vi "Arm Control.vi"(9 "Position":dbl, 10 "Arm Target":string) -> ()   [LabVIEW 2020]
uses:
  <vilib>/addons/control/pid/NI_PID_pid.lvlib
  <vilib>/addons/control/pid/pid.llb/PID (DBL).vi
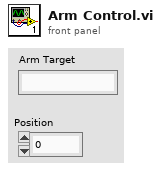
[diagram p1: front panel]
types:
  T1 = cluster{"proportional gain (Kc)":dbl, "integral time (Ti, min)":dbl, "derivative time (Td, min)":dbl}
  T2 = typedef "WPI_MotorControlDeviceRef.ctl" = cluster{"DeviceStatus":errorcluster, "Type":T3, "PWM":cluster{"PWM Channel":T4, "DeadBand":T5}, "CAN":cluster{"Device Number":u8, "SetOutput VI Ref":variant, "GetOutput VI Ref":variant, "Enable VI Ref":variant, "Disable VI Ref":variant, "Data":variant}, "Invert":bool, "DIO PWM":cluster{"PWM \"Enable\" Channel":T4, "DIOChannel":T6, "PWM Rate":dbl}}
  T3 = typedef "WPI_MotorControlType.ctl" = enum16{"PWM", "CAN", "DIO PWM"}
  T4 = typedef "FPGA_DIOPWMChannel.ctl" = enum8{"PWM 0", "PWM 1", "PWM 2", "PWM 3", "PWM 4", "PWM 5", "PWM 6", "PWM 7", "PWM 8", "PWM 9", "PWM MXP 0", "PWM MXP 1", "PWM MXP 2", "PWM MXP 3", "PWM MXP 4", "PWM MXP 5", "PWM MXP 6", "PWM MXP 7", "PWM MXP 8", "PWM MXP 9", "Invalid"}
  T5 = typedef "WPI_PWMDeadband.ctl" = cluster{"Name":string, "maxPositivePwm":i32, "minPositivePwm":i32, "centerPwm":i32, "maxNegativePwm":i32, "minNegativePwm":i32, "angularRange":u16}
  T6 = typedef "FPGA_DIOChannel.ctl" = enum8{"DIO 0", "DIO 1", "DIO 2", "DIO 3", "DIO 4", "DIO 5", "DIO 6", "DIO 7", "DIO 8", "DIO 9", "DIO MXP 0", "DIO MXP 1", "DIO MXP 2", "DIO MXP 3", "DIO MXP 4", "DIO MXP 5", "DIO MXP 6", "DIO MXP 7", "DIO MXP 8", "DIO MXP 9", "DIO MXP 10", "DIO MXP 11", "DIO MXP 12", "DIO MXP 13", "DIO MXP 14", "DIO MXP 15", "SPI Port CS1", "SPI Port CS2", "SPI Port CS3", "SPI Port MISO", "SPI Port MOSI", "Invalid"}
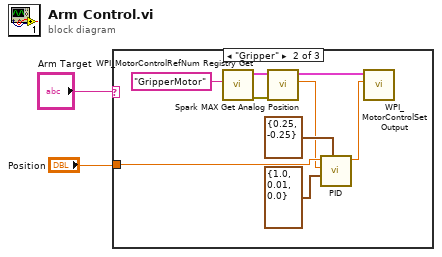
[diagram p0: block diagram]
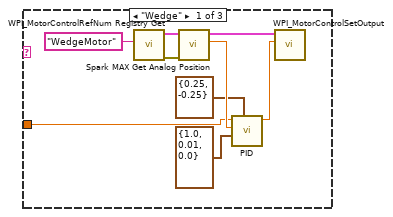
[diagram p2: hidden frame]
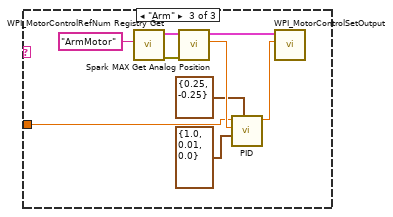
[diagram p3: hidden frame]
diagram:
  n1 = case shown="\"Gripper\"" "Arm Target" {
    tunnel: "Position" -> [w3 w20 w21]
    frame "Wedge" {
      n2 = call <vilib>:"WPI_MotorControlRefNum Registry Get.vi"("refnum name"="WedgeMotor") -> ("error out"=w8:errorcluster, "MotorControlDevRef"=w7:T2)  [unwired: 9 in]
      n3 = call <vilib>:"Spark MAX Get Analog Position.vi"("error in (no error)"=w8, "MotorControlDevRef in"=w7) -> ("Analog Position"=w9:dbl, "MotorControlDevRef out"=w10:T2)  [unwired: 6 in, 2 out]
      n4 = call-poly <vilib>:"PID.vi"("output range"=cluster{"output high":dbl, "output low":dbl} {"output high"=0.25, "output low"=-0.25}, "PID gains"=T1 {"proportional gain (Kc)"=1.0, "integral time (Ti, min)"=0.01, "derivative time (Td, min)"=0.0}, "process variable"=w9, "setpoint"=w3) -> ("output"=w11:dbl)  [unwired: 6 in, 1 out]
      n5 = call <vilib>:"WPI_MotorControlSetOutput.vi"("Output"=w11, "MotorControlDevRef"=w10) -> ()  [unwired: 7 in, 3 out]
    }
    frame "Gripper" {
      n6 = call <vilib>:"WPI_MotorControlRefNum Registry Get.vi"("refnum name"="GripperMotor") -> ("error out"=w15:errorcluster, "MotorControlDevRef"=w17:T2)  [unwired: 9 in]
      n7 = call <vilib>:"Spark MAX Get Analog Position.vi"("error in (no error)"=w15, "MotorControlDevRef in"=w17) -> ("Analog Position"=w14:dbl, "MotorControlDevRef out"=w13:T2)  [unwired: 6 in, 2 out]
      n8 = call-poly <vilib>:"PID.vi"("output range"=cluster{"output high":dbl, "output low":dbl} {"output high"=0.25, "output low"=-0.25}, "PID gains"=T1 {"proportional gain (Kc)"=1.0, "integral time (Ti, min)"=0.01, "derivative time (Td, min)"=0.0}, "process variable"=w14, "setpoint"=w20) -> ("output"=w12:dbl)  [unwired: 6 in, 1 out]
      n9 = call <vilib>:"WPI_MotorControlSetOutput.vi"("Output"=w12, "MotorControlDevRef"=w13) -> ()  [unwired: 7 in, 3 out]
    }
    frame "Arm" {
      n10 = call <vilib>:"WPI_MotorControlRefNum Registry Get.vi"("refnum name"="ArmMotor") -> ("error out"=w26:errorcluster, "MotorControlDevRef"=w25:T2)  [unwired: 9 in]
      n11 = call <vilib>:"Spark MAX Get Analog Position.vi"("error in (no error)"=w26, "MotorControlDevRef in"=w25) -> ("Analog Position"=w27:dbl, "MotorControlDevRef out"=w28:T2)  [unwired: 6 in, 2 out]
      n12 = call-poly <vilib>:"PID.vi"("output range"=cluster{"output high":dbl, "output low":dbl} {"output high"=0.25, "output low"=-0.25}, "PID gains"=T1 {"proportional gain (Kc)"=1.0, "integral time (Ti, min)"=0.01, "derivative time (Td, min)"=0.0}, "process variable"=w27, "setpoint"=w21) -> ("output"=w29:dbl)  [unwired: 6 in, 1 out]
      n13 = call <vilib>:"WPI_MotorControlSetOutput.vi"("Output"=w29, "MotorControlDevRef"=w28) -> ()  [unwired: 7 in, 3 out]
    }
  }
